vi "Create file path.vi"(4 "MASTER in":T1 {"Image data"."Color Palette" items=["Grayscale U8", "False Color", "Overexposed"]; "Image data"."Exposure time [us]" format="%#_10g"; "Queue"."Initial time [s]" format="%_19f"; "Queue"."Raw data [V]\n(all samples)" format="%0.2f"; "Queue"."Timestamp [s]" format="%_19f"}) -> (1 "MASTER out":T1 {"Image data"."Color Palette" items=["Grayscale U8", "False Color", "Overexposed"]; "Image data"."Exposure time [us]" format="%#_10g"; "Queue"."Initial time [s]" format="%_19f"; "Queue"."Raw data [V]\n(all samples)" format="%0.2f"; "Queue"."Timestamp [s]" format="%_19f"})   [LabVIEW 2020]
uses:
  MASTER.ctl
  Constants.ctl
  QBundle.ctl
  Queue.ctl
  Image data.ctl
  <vilib>/userdefined/High Color/IMAQdx.ctl
  <vilib>/vision/Image Controls.llb/IMAQ Image.ctl
  Image QBundle.ctl
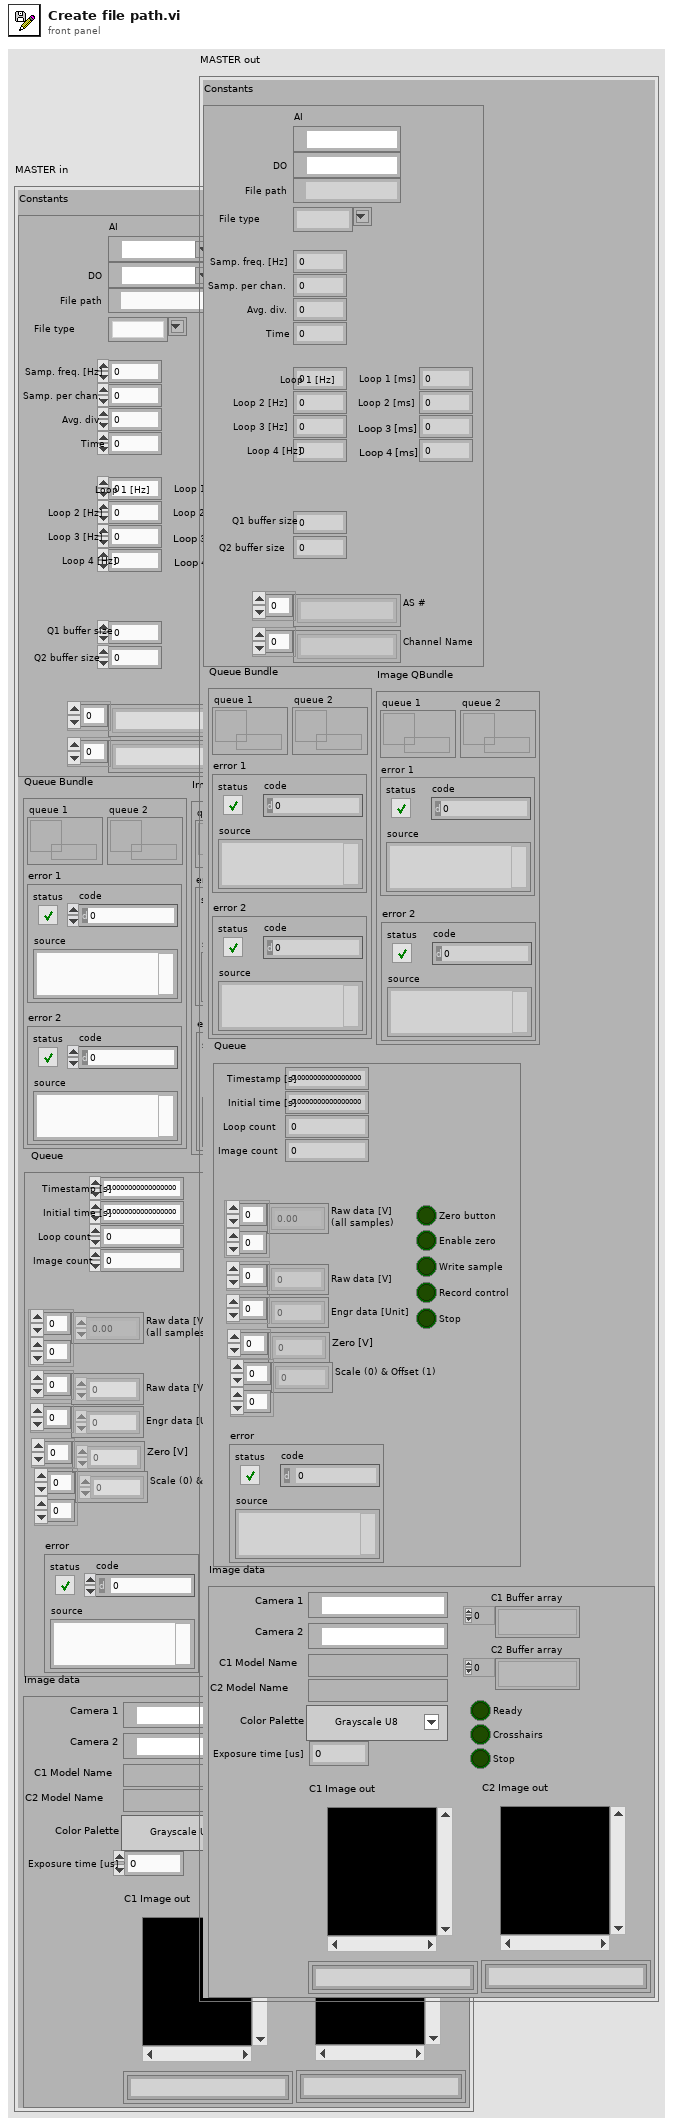
[diagram p1: front panel]
types:
  T1 = typedef "MASTER.ctl" = cluster{"Constants":T2, "Queue Bundle":T3, "Queue":T4, "Image data":T5, "Image QBundle ":T8}
  T2 = typedef "Constants.ctl" = cluster{"Time":u16, "Samp. freq. [Hz]":dbl, "Samp. per chan.":i32, "Avg. div.":i32, "File path":path, "AI":refnum<k21>, "Loop 1 [Hz]":dbl, "Loop 2 [Hz]":dbl, "Loop 3 [Hz]":dbl, "Loop 1 [ms]":dbl, "Loop 2 [ms]":dbl, "Loop 3 [ms]":dbl, "Q1 buffer size":i32, "Q2 buffer size":i32, "File type":string, "Loop 4 [Hz]":dbl, "Loop 4 [ms]":dbl, "Channel Name":string[], "AS #":string[], "DO":refnum<k21>}
  T3 = typedef "QBundle.ctl" = cluster{"queue 1":refnum<queue>, "error 1":errorcluster, "queue 2":refnum<queue>, "error 2":errorcluster}
  T4 = typedef "Queue.ctl" = cluster{"Enable zero":bool, "Engr data [Unit]":dbl[], "Zero button":bool, "Zero [V]":dbl[], "Timestamp [s]":dbl, "Write sample":bool, "Record control":bool, "Stop":bool, "error":errorcluster, "Raw data [V]\n(all samples)":dbl[][], "Raw data [V]":dbl[], "Loop count":i64, "Initial time [s]":dbl, "Scale (0) & Offset (1)":dbl[][], "Image count":dbl}
  T5 = typedef "Image data.ctl" = cluster{"Camera 1":T6, "Camera 2":T6, "C1 Image out ":T7, "C2 Image out":T7, "C1 Model Name":string, "C2 Model Name":string, "Exposure time [us]":dbl, "Color Palette":u16, "C1 Buffer array":T7[], "Ready":bool, "C2 Buffer array":T7[], "Crosshairs":bool, "Stop":bool}
  T6 = typedef "IMAQdx.ctl" = refnum<k21>
  T7 = typedef "IMAQ Image.ctl" = refnum<image>
  T8 = typedef "Image QBundle.ctl" = cluster{"queue 1":refnum<queue>, "error 1":errorcluster, "queue 2":refnum<queue>, "error 2":errorcluster}
  T9 = enum16{"open", "replace", "create", "open or create", "replace or create", "replace or create with confirmation"}
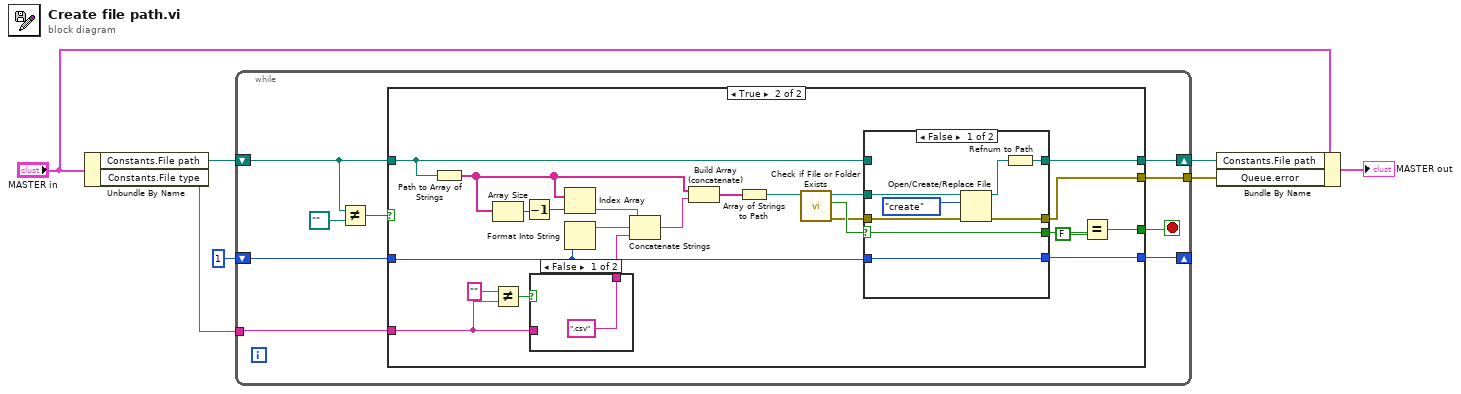
[diagram p0: block diagram]
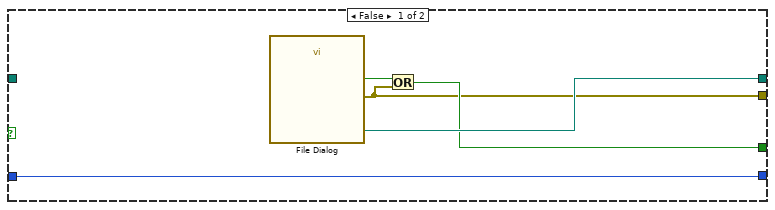
[diagram p2: hidden frame]
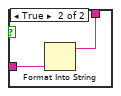
[diagram p3: hidden frame]
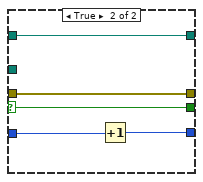
[diagram p4: hidden frame]
diagram:
  n1 = Unbundle By Name("MASTER in") -> ("Constants.File path"=w5:path, "Constants.File type"=w2:string)
  n2 = while {
    tunnel: w2 -> [w16]
    shift-right: [w15] -> w4
    shift-left: w5 -> [w11]
    shift-right: [w9] -> _
    shift-left: 1 ("Num") -> [w10]
    tunnel: [w8] -> w1
    stop <- w12 stop-if-true
    n3 = Not Equal?(x=w11, y=path "") -> (x != y?=w14:bool)
    n4 = case shown="True" w14 {
      tunnel: w16 -> [_ w25]
      tunnel: w11 -> [_ w28]
      tunnel: [w21 w33] -> w15
      tunnel: [w18 w31] -> w12
      tunnel: w10 -> [w20 w27]
      tunnel: [w20 w32] -> w9
      tunnel: [w17 w22] -> w8
      frame False {
        n5 = call "File Dialog"() -> ("selected path"=w21:path, "cancelled"=w19:bool, "error out"=w17:errorcluster)  [unwired: 12 in, 1 out]
        n6 = Or(x=w19, y=w17) -> (x .or. y?=w18:bool)
      }
      frame True {
        n7 = Path to Array of Strings(0:w28) -> (2:w37:string[])  [unwired: 1 out]
        n8 = Array Size(array=w37) -> (size(s)=w40:i32)
        n9 = Not Equal?(x="", y=w25) -> (x != y?=w26:bool)
        n10 = Decrement(x=w40) -> (x-1=w41:i32)
        n11 = case shown="False" w26 {
          tunnel: [".csv" w47] -> w43
          tunnel: w25 -> [_ w46]
          frame False {
          }
          frame True {
            n12 = Format Into String(w46) -> (resulting string=w47:string)  [unwired: 3 in, 1 out]
          }
        }
        n13 = Index Array(array=w37, index=w41) -> (element=w42:string)
        n14 = Format Into String(w27) -> (resulting string=w38:string)  [unwired: 3 in, 1 out]
        n15 = Concatenate Strings(w42, w38, w43) -> (w39:string)
        n16 = Build Array (concatenate)(w37, w39) -> (w44:string[])
        n17 = Array of Strings to Path(0:w44) -> (2:w36:path)  [unwired: 1 in]
        n18 = call <vilib>:"Check if File or Folder Exists.vi"("path"=w36) -> ("error out"=w23:errorcluster, "file or folder exists?"=w34:bool, "dup path"=w35:path)  [unwired: 8 in]
        n19 = case shown="False" w34 {
          selector: w34 -> [w52 w59]
          tunnel: w35 -> [w54 _]
          tunnel: [w50 w57] -> w33
          tunnel: [w51 w58] -> w32
          tunnel: w27 -> [w51 w60]
          tunnel: [w52 w59] -> w30
          tunnel: w28 -> [_ w57]
          tunnel: w23 -> [w49 w56]
          tunnel: [w48 w56] -> w22
          frame False {
            n20 = Open/Create/Replace File(file path (use dialog)=w54, error in=w49, operation (0:open)=T9."create") -> (refnum out=w53:refnum<file>, error out=w48:errorcluster)  [unwired: 3 in, 1 out]
            n21 = Refnum to Path(1:w53) -> (0:w50:path)
          }
          frame True {
            n22 = Increment(x=w60) -> (x+1=w58:i32)
          }
        }
        n23 = Equal?(x=w30, y=FALSE) -> (x = y?=w31:bool)
      }
    }
  }
  n24 = Bundle By Name(cluster="MASTER in", "Constants.File path"=w4, "Queue.error"=w1) -> (→"MASTER out":T1)
